vi "sushu-the first greater than 0 after less than 0.vi"(6 "Choose":string(combo)="Less", 7 "Direction":string(combo)="Forward", 8 "error out":errorcluster, 11 "Array In":dbl[](array[numeric])) -> (0 "error out 2":errorcluster)   [LabVIEW 2021]
panel:
  in  "OK":bool
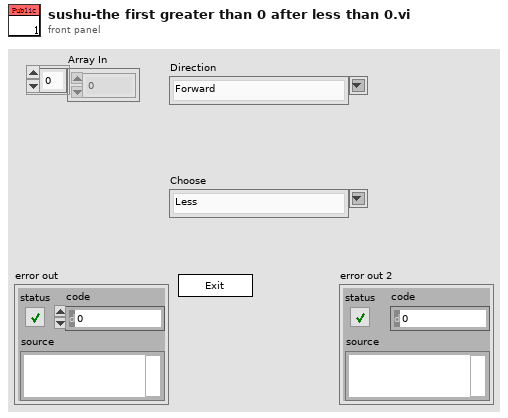
[diagram p1: front panel]
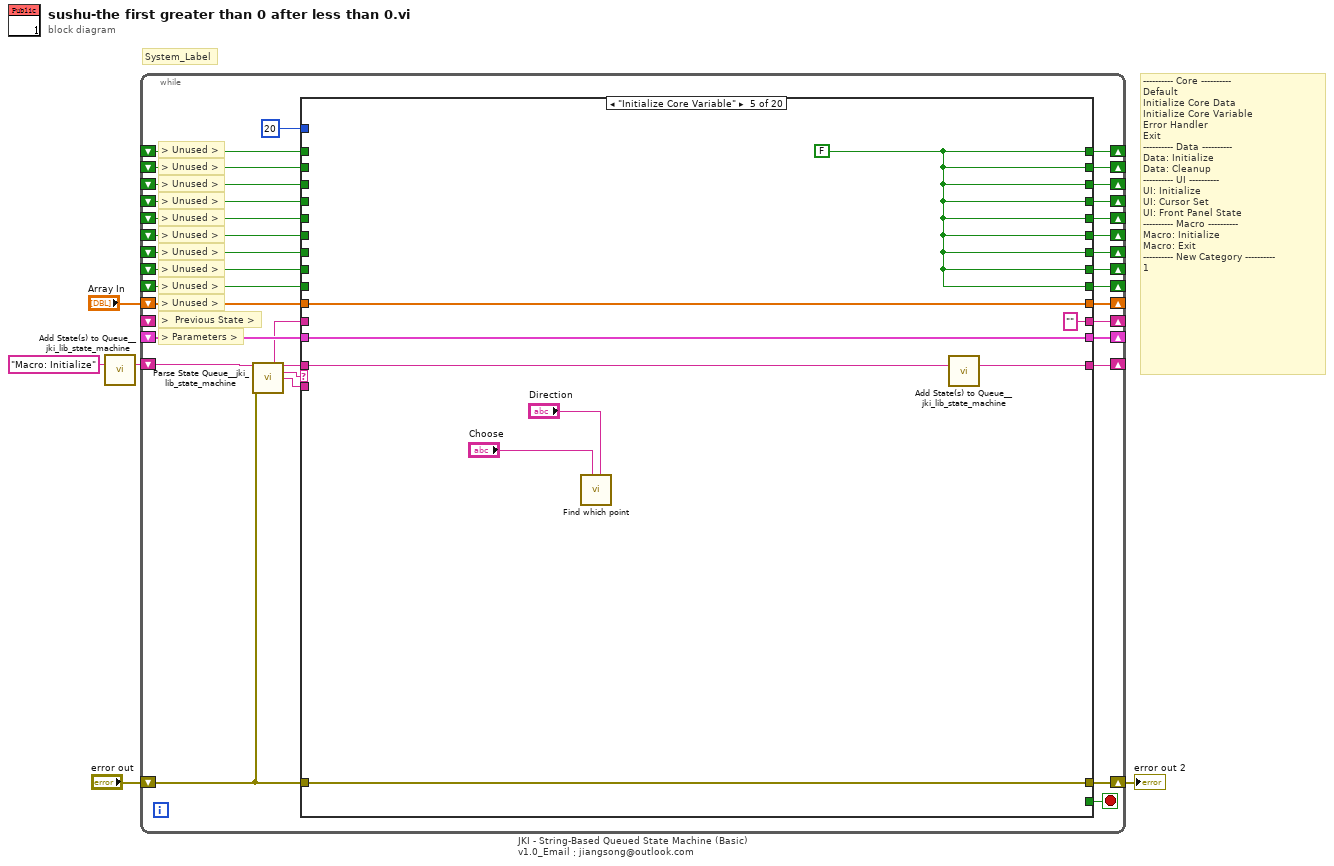
[diagram p0: block diagram]
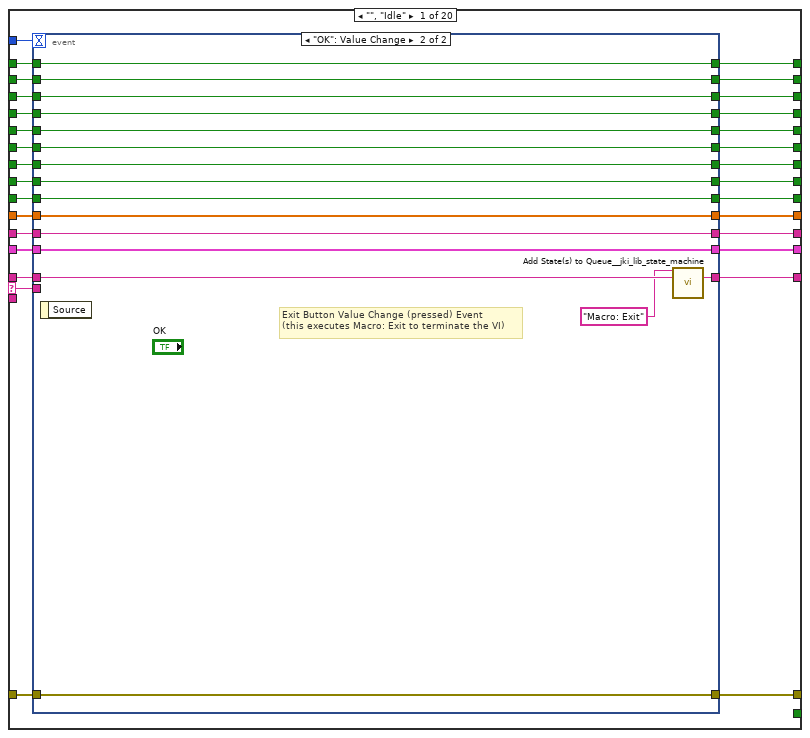
[diagram p2: hidden frame]
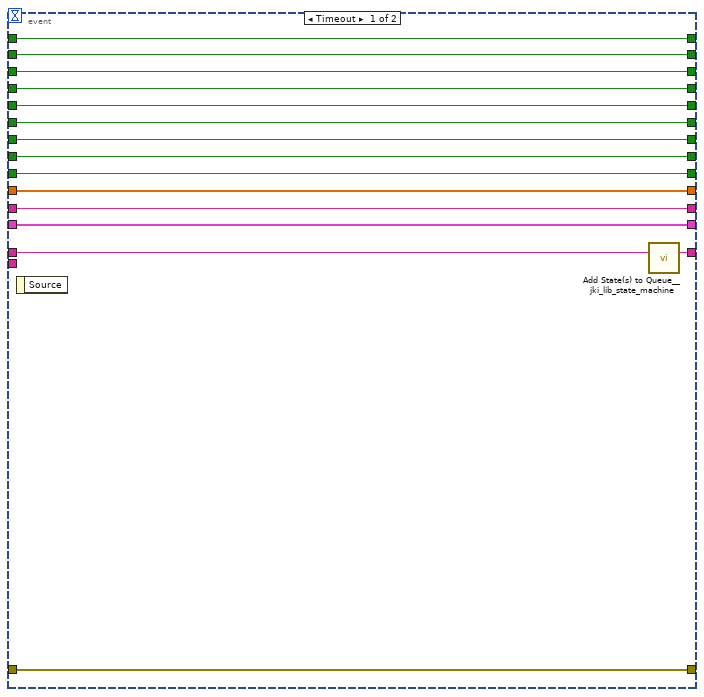
[diagram p3: hidden frame]
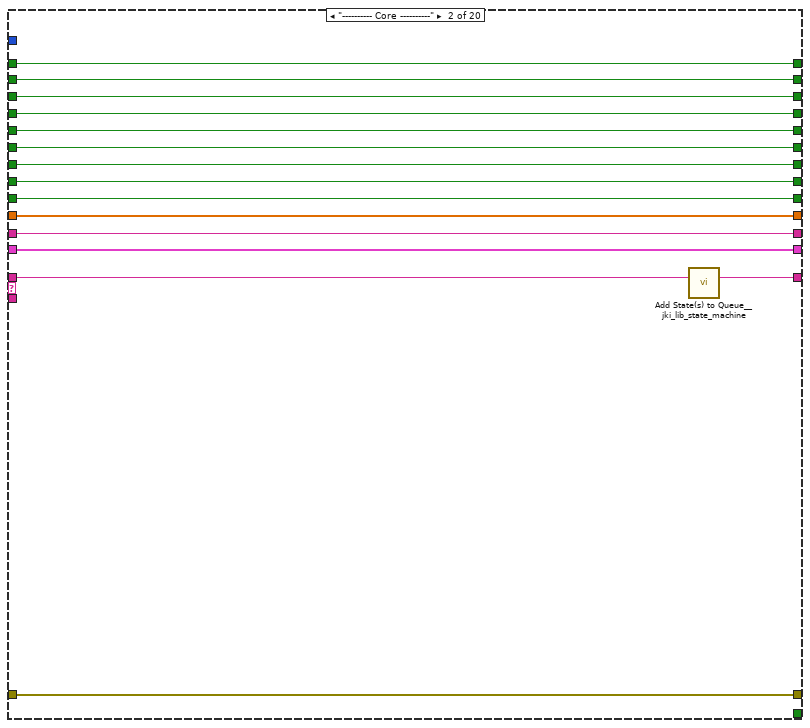
[diagram p4: hidden frame]
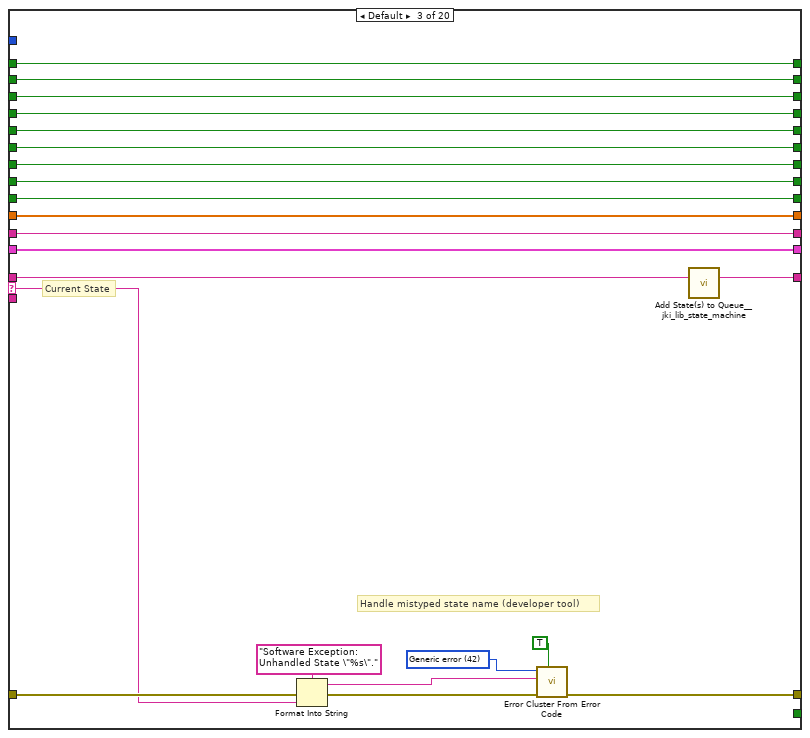
[diagram p5: hidden frame]
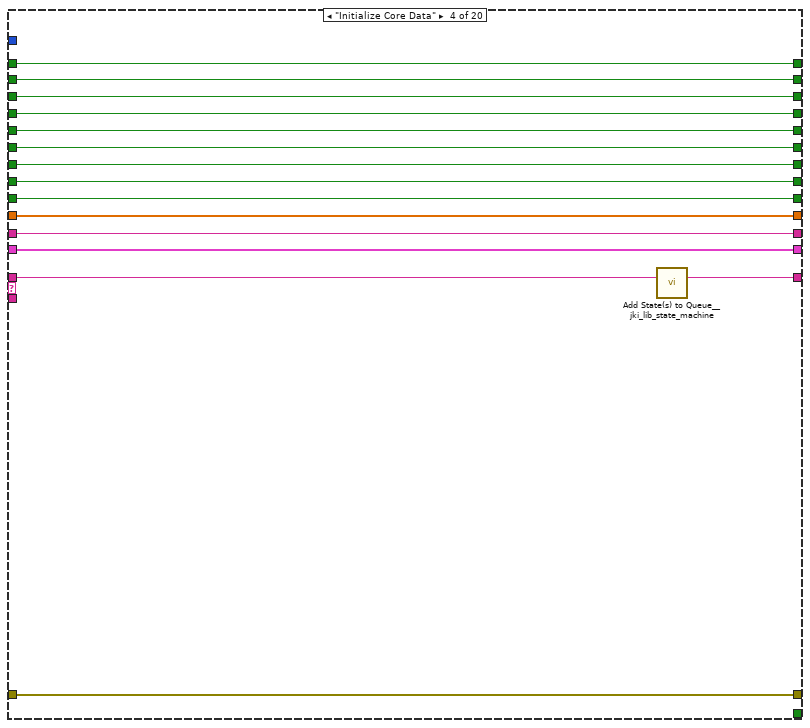
[diagram p6: hidden frame]
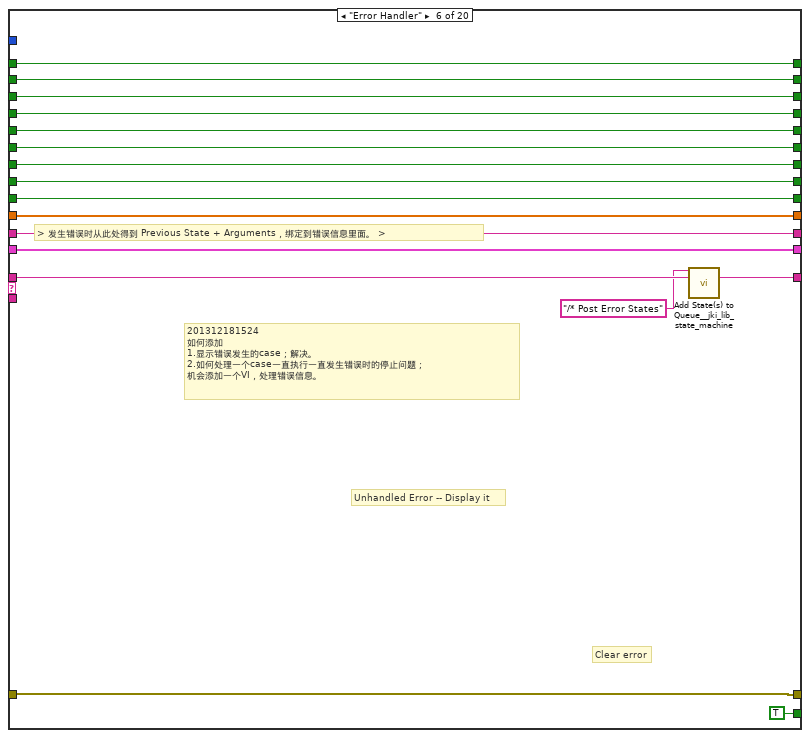
[diagram p7: hidden frame]
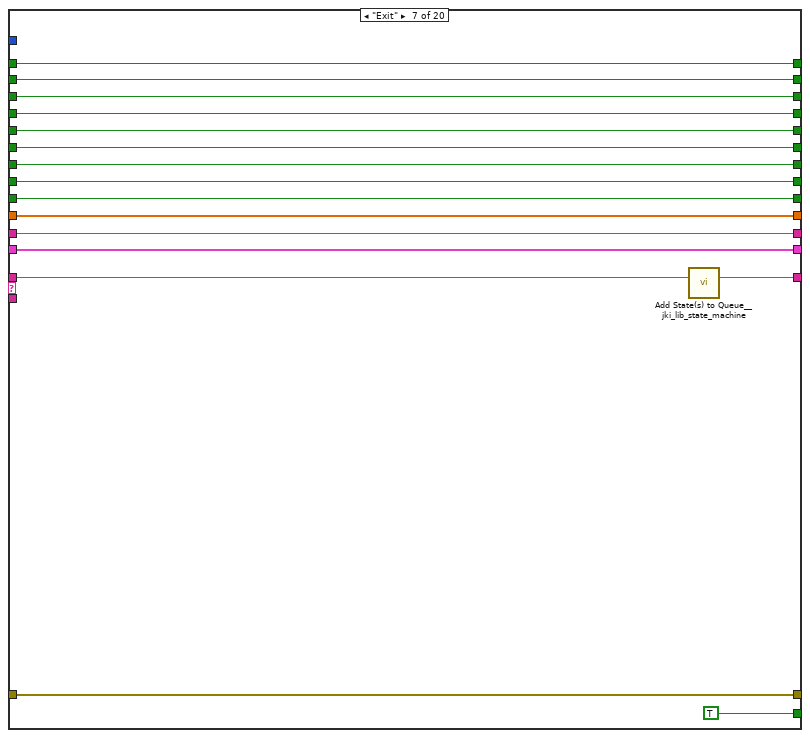
[diagram p8: hidden frame]
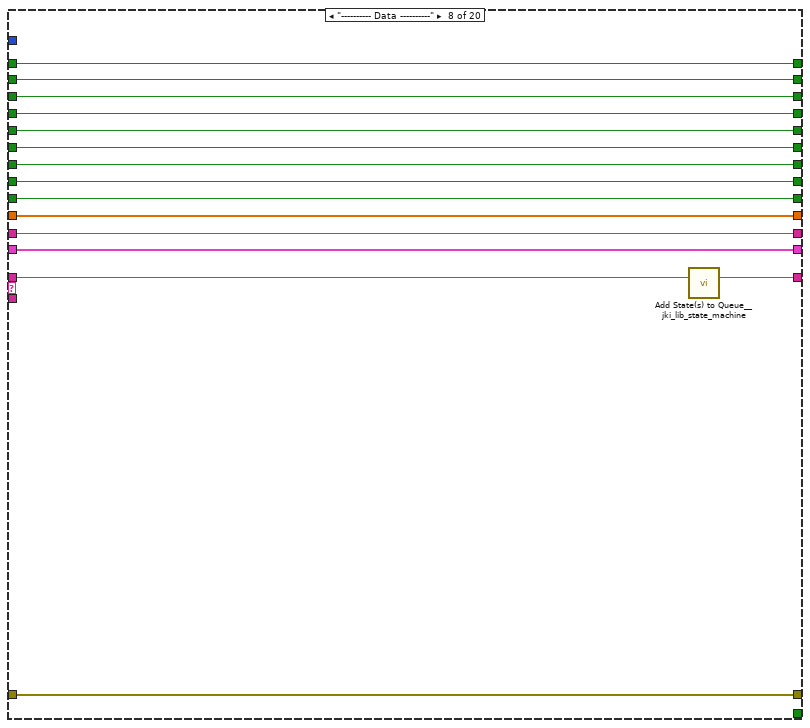
[diagram p9: hidden frame]
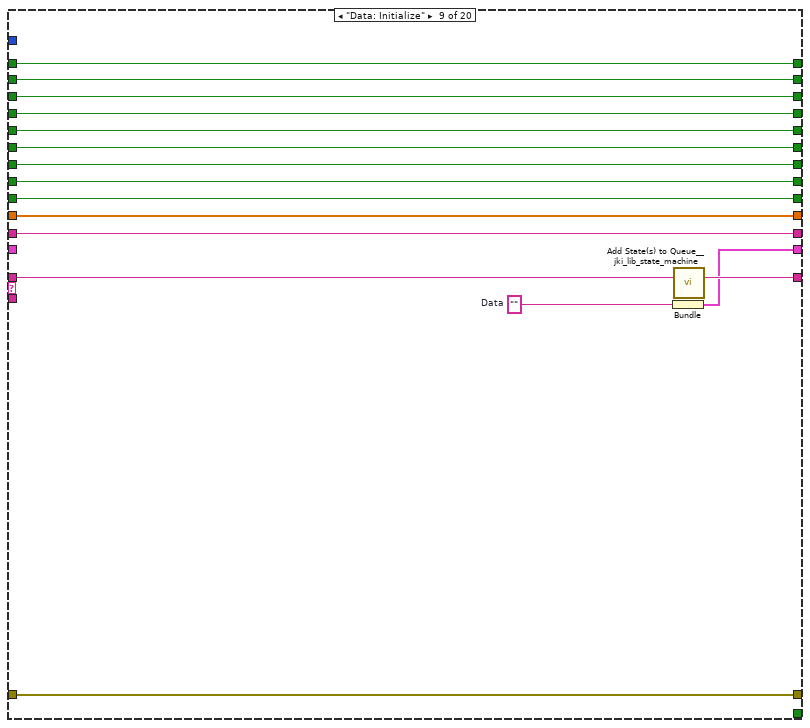
[diagram p10: hidden frame]
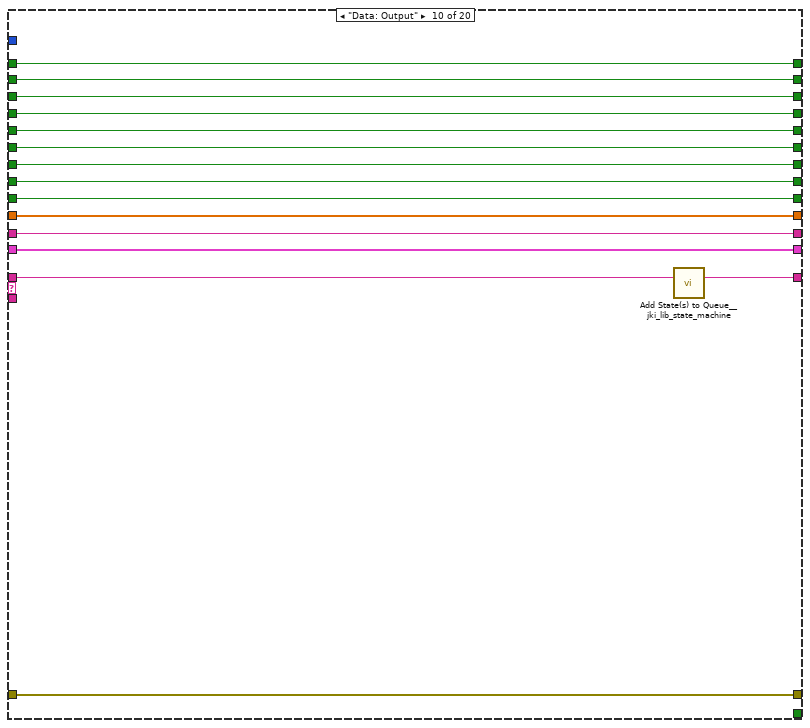
[diagram p11: hidden frame]
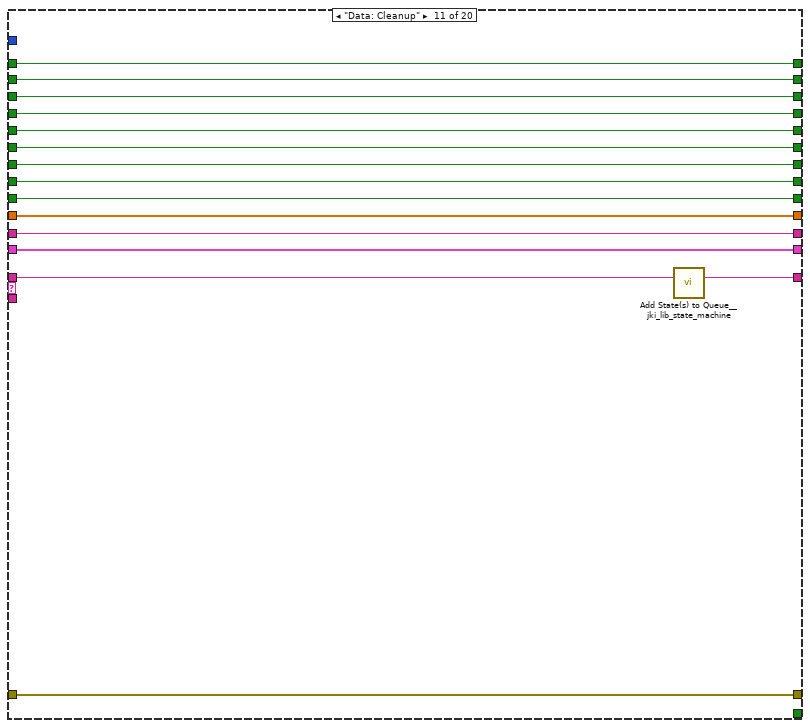
[diagram p12: hidden frame]
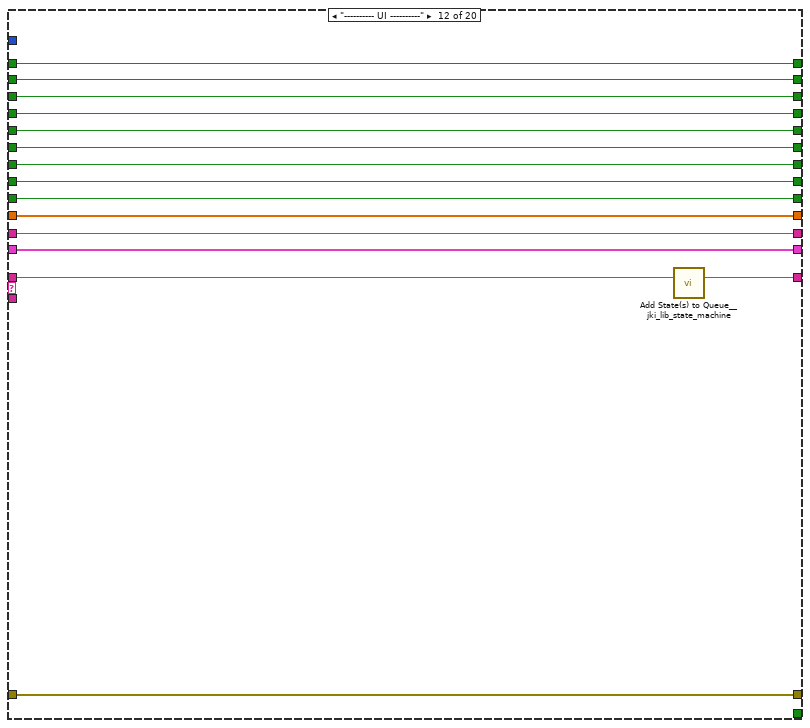
[diagram p13: hidden frame]
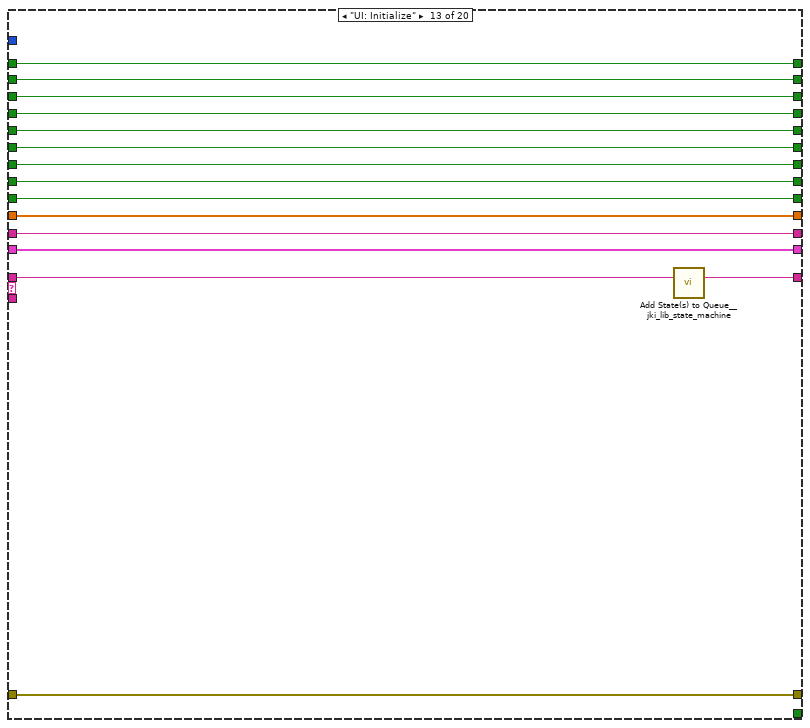
[diagram p14: hidden frame]
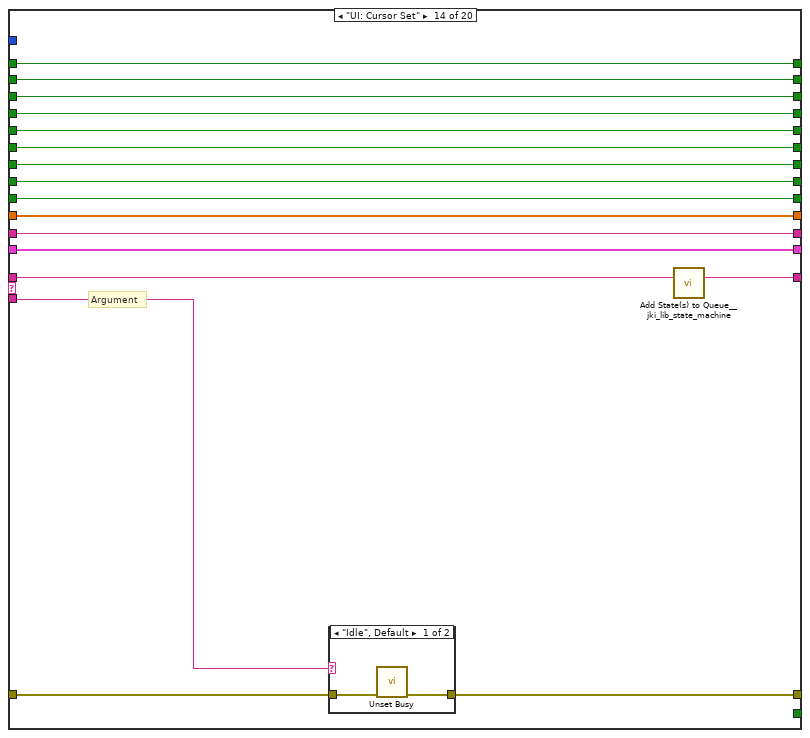
[diagram p15: hidden frame]
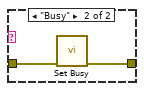
[diagram p16: hidden frame]
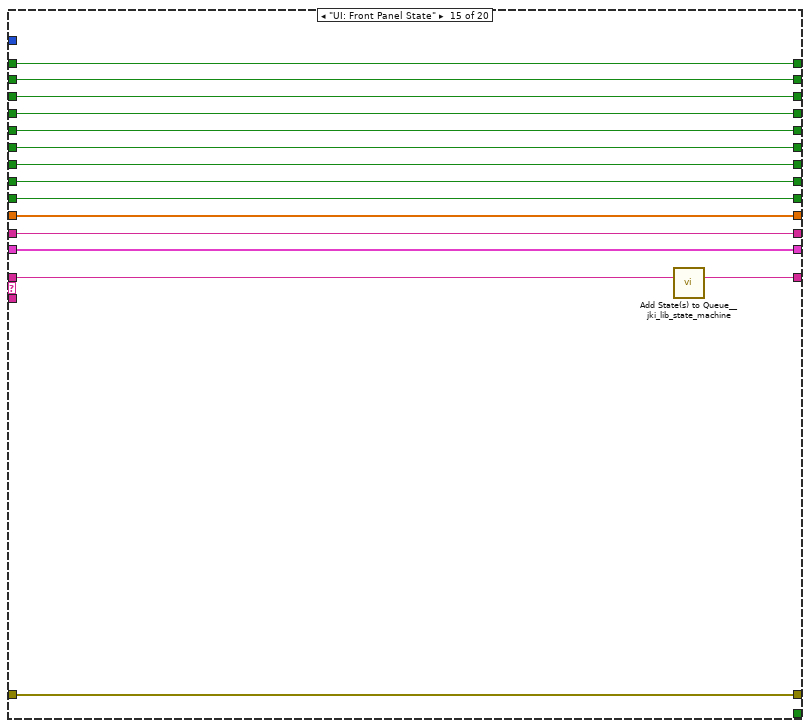
[diagram p17: hidden frame]
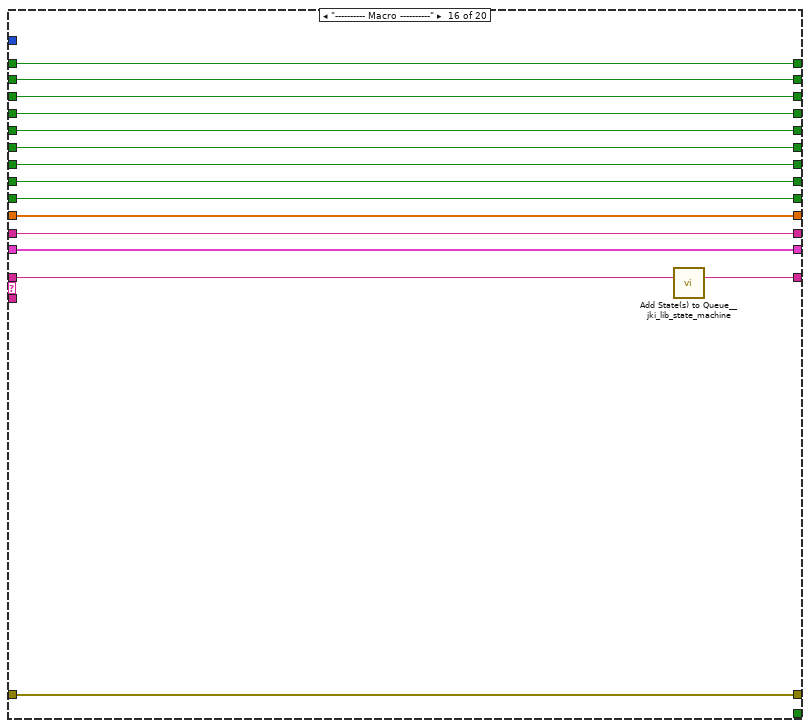
[diagram p18: hidden frame]
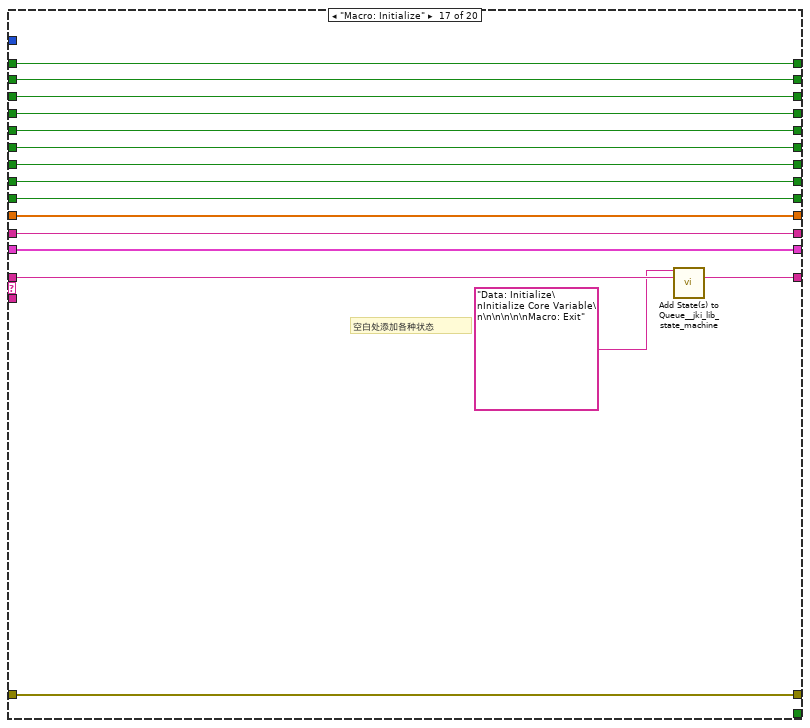
[diagram p19: hidden frame]
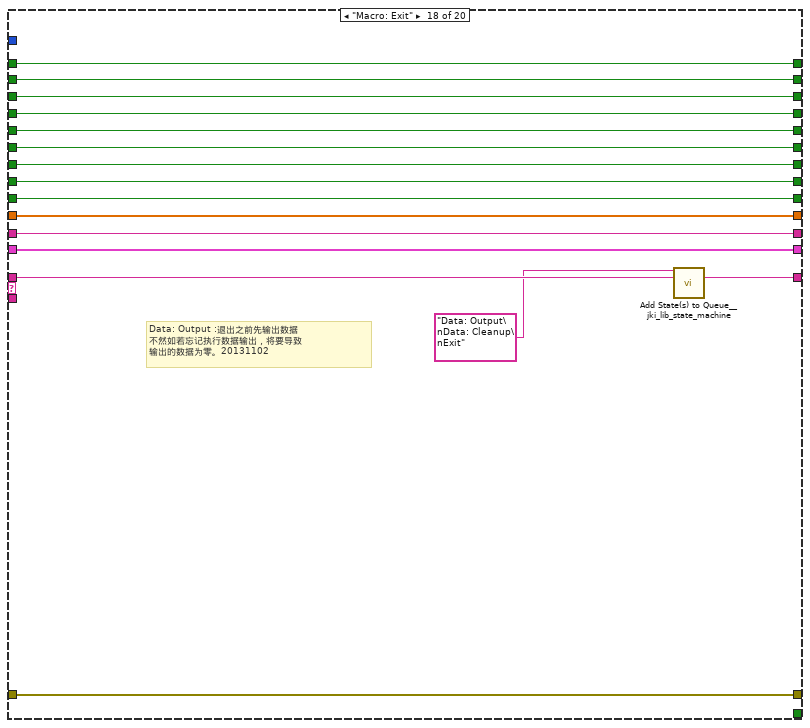
[diagram p20: hidden frame]
diagram:
  # "---------- Core ----------\nDefault\nInitialize Core Data\nInitialize Core Variable\nError Handler\nExit\n---------- Data ----------\nData: Initialize\nData: Cleanup\n---------- UI ----------\nUI: Initialize\nUI: Cursor Set\nUI: Front Panel State\n---------- Macro ----------\nMacro: Initialize\nMacro: Exit\n---------- New Category ----------\n1"
  # "System_Label"
  n1 = call <vilib>:"Add State(s) to Queue__jki_lib_state_machine.vi"("State(s) in (\"\")"="Macro: Initialize") -> ("States Out"=w3:string)  [unwired: 14 in]
  n2 = while "JKI - String-Based Queued State Machine (Basic) v1.0_Email：jiangsong@outlook.com" {
    shift-right: [w34] -> w5
    shift-left: "error out" -> [w30]
    shift-right: [w33] -> _
    shift-left: w3 -> [w35]
    shift-right: [w29] -> _
    shift-left: _ -> [w28]
    shift-right: [w16] -> _
    shift-left: _ -> [w24]
    shift-right: [w17] -> _
    shift-left: _ -> [w25]
    shift-right: [w18] -> _
    shift-left: _ -> [w26]
    shift-right: [w19] -> _
    shift-left: _ -> [w27]
    shift-right: [w12] -> _
    shift-left: _ -> [w20]
    shift-right: [w13] -> _
    shift-left: _ -> [w21]
    shift-right: [w14] -> _
    shift-left: _ -> [w22]
    shift-right: [w15] -> _
    shift-left: _ -> [w23]
    shift-right: [w7] -> _
    shift-left: _ -> [w10]
    shift-right: [w8] -> _
    shift-left: _ -> [_]
    shift-right: [w9] -> _
    shift-left: "Array In" -> [w11]
    stop <- w32 stop-if-true
    # "> Parameters >"
    # ">  Previous State >"
    # "> Unused >"
    # "> Unused >"
    # "> Unused >"
    # "> Unused >"
    # "> Unused >"
    # "> Unused >"
    # "> Unused >"
    # "> Unused >"
    # "> Unused >"
    # "> Unused >"
    n3 = call <vilib>:"Parse State Queue__jki_lib_state_machine.vi"("State Queue"=w35, "Error In (no error)"=w30) -> ("Previous State"=w6:string, "Remaining States"=w37:string, "Current State"=w38:string, "Arguments"=w36:string)  [unwired: 10 in]
    n4 = case shown="\"Initialize Core Variable\"" w38 {
      selector: w38 -> [w39 _ w115 _ _ _ _ _ _ _ _ _ _ _ _ _ _ _ _ _]
      tunnel: w37 -> [w68 w114 w136 w151 w160 w177 w193 w208 w224 w239 w254 w269 w284 w301 w320 w335 w351 w367 w382 w397]
      tunnel: w36 -> [_ _ _ _ _ _ _ _ _ _ _ _ _ w288 _ _ _ _ _ _]
      tunnel: [w66 w112 w116 w139 w158 w161 w179 w195 w212 w227 w241 w256 w271 w286 w307 w322 w338 w355 w370 w385] -> w34
      tunnel: w30 -> [w65 w112 w117 w139 w158 w161 w179 w195 w212 w227 w241 w256 w271 w287 w307 w322 w338 w355 w370 w385]
      tunnel: [w67 w113 w135 w150 w159 w176 w192 w207 w223 w238 w253 w268 w283 w300 w319 w334 w350 w366 w381 w396] -> w33
      tunnel: [_ _ _ _ _ TRUE TRUE _ _ _ _ _ _ _ _ _ _ _ _ _] -> w32
      tunnel: 20 ("Timeout") -> [w64 _ _ _ _ _ _ _ _ _ _ _ _ _ _ _ _ _ _ _]
      tunnel: [w63 w111 w134 w149 w154 w175 w191 w206 w222 w237 w252 w267 w282 w299 w318 w333 w349 w365 w380 w395] -> w29
      tunnel: w28 -> [w62 w111 w134 w149 _ w175 w191 w206 w222 w237 w252 w267 w282 w299 w318 w333 w349 w365 w380 w395]
      tunnel: w27 -> [w61 w110 w133 w148 _ w174 w190 w205 w221 w236 w251 w266 w281 w298 w317 w332 w348 w364 w379 w394]
      tunnel: w26 -> [w60 w109 w132 w147 _ w173 w189 w204 w220 w235 w250 w265 w280 w297 w316 w331 w347 w363 w378 w393]
      tunnel: w25 -> [w59 w108 w131 w146 _ w172 w188 w203 w219 w234 w249 w264 w279 w296 w315 w330 w346 w362 w377 w392]
      tunnel: w24 -> [w58 w107 w130 w145 _ w171 w187 w202 w218 w233 w248 w263 w278 w295 w314 w329 w345 w361 w376 w391]
      tunnel: w23 -> [w57 w106 w129 w144 _ w170 w186 w201 w217 w232 w247 w262 w277 w294 w313 w328 w344 w360 w375 w390]
      tunnel: w22 -> [w56 w105 w128 w143 _ w169 w185 w200 w216 w231 w246 w261 w276 w293 w312 w327 w343 w359 w374 w389]
      tunnel: w21 -> [w55 w104 w127 w142 _ w168 w184 w199 w215 w230 w245 w260 w275 w292 w311 w326 w342 w358 w373 w388]
      tunnel: w20 -> [w54 w103 w126 w141 _ w167 w183 w198 w214 w229 w244 w259 w274 w291 w310 w325 w341 w357 w372 w387]
      tunnel: [w53 w110 w133 w148 w154 w174 w190 w205 w221 w236 w251 w266 w281 w298 w317 w332 w348 w364 w379 w394] -> w19
      tunnel: [w52 w109 w132 w147 w154 w173 w189 w204 w220 w235 w250 w265 w280 w297 w316 w331 w347 w363 w378 w393] -> w18
      tunnel: [w51 w108 w131 w146 w154 w172 w188 w203 w219 w234 w249 w264 w279 w296 w315 w330 w346 w362 w377 w392] -> w17
      tunnel: [w50 w107 w130 w145 w154 w171 w187 w202 w218 w233 w248 w263 w278 w295 w314 w329 w345 w361 w376 w391] -> w16
      tunnel: [w49 w106 w129 w144 w154 w170 w186 w201 w217 w232 w247 w262 w277 w294 w313 w328 w344 w360 w375 w390] -> w15
      tunnel: [w48 w105 w128 w143 w154 w169 w185 w200 w216 w231 w246 w261 w276 w293 w312 w327 w343 w359 w374 w389] -> w14
      tunnel: [w47 w104 w127 w142 w154 w168 w184 w199 w215 w230 w245 w260 w275 w292 w311 w326 w342 w358 w373 w388] -> w13
      tunnel: [w46 w103 w126 w141 w154 w167 w183 w198 w214 w229 w244 w259 w274 w291 w310 w325 w341 w357 w372 w387] -> w12
      tunnel: w11 -> [w44 w102 w125 w140 w155 w166 w182 w197 w213 w228 w243 w258 w273 w290 w309 w324 w340 w356 w371 w386]
      tunnel: w6 -> [w42 w100 w124 w137 _ w163 w178 w194 w209 w225 w240 w255 w270 w285 w306 w321 w336 w352 w368 w383]
      tunnel: w10 -> [w40 w101 w123 w138 w157 w165 w181 w196 _ w226 w242 w257 w272 w289 w308 w323 w339 w354 w369 w384]
      tunnel: [w45 w102 w125 w140 w155 w166 w182 w197 w213 w228 w243 w258 w273 w290 w309 w324 w340 w356 w371 w386] -> w9
      tunnel: [w43 w100 w124 w137 "" ("Previous State + Arguments") w163 w178 w194 w209 w225 w240 w255 w270 w285 w306 w321 w336 w352 w368 w383] -> w8
      tunnel: [w41 w101 w123 w138 w157 w165 w181 w196 w211 w226 w242 w257 w272 w289 w308 w323 w339 w354 w369 w384] -> w7
      frame "", "Idle" {
        n5 = event shown="[1] \"OK\": Value Change" {
          selector: _ -> [_ _]
          dyn-events: _ -> [_ _]
          timeout: w64 -> [_ _]
          tunnel: w68 -> [w83 w99]
          tunnel: [w82 w98] -> w67
          tunnel: [w81 w97] -> w66
          tunnel: w65 -> [w81 w97]
          tunnel: [w80 w96] -> w63
          tunnel: w62 -> [w80 w96]
          tunnel: w61 -> [w79 w95]
          tunnel: w60 -> [w78 w94]
          tunnel: w59 -> [w77 w93]
          tunnel: w58 -> [w76 w92]
          tunnel: w57 -> [w75 w91]
          tunnel: w56 -> [w74 w90]
          tunnel: w55 -> [w73 w89]
          tunnel: w54 -> [w72 w88]
          tunnel: [w79 w95] -> w53
          tunnel: [w78 w94] -> w52
          tunnel: [w77 w93] -> w51
          tunnel: [w76 w92] -> w50
          tunnel: [w75 w91] -> w49
          tunnel: [w74 w90] -> w48
          tunnel: [w73 w89] -> w47
          tunnel: [w72 w88] -> w46
          tunnel: [w71 w87] -> w45
          tunnel: w44 -> [w71 w87]
          tunnel: [w69 w84] -> w43
          tunnel: w42 -> [w69 w84]
          tunnel: [w70 w86] -> w41
          tunnel: w40 -> [w70 w86]
          tunnel: w39 -> [_ _]
          event Timeout {
            n6 = event-data() -> ()  [unwired: 1 in, 1 out]
            n7 = call <vilib>:"Add State(s) to Queue__jki_lib_state_machine.vi"("State(s) in (\"\")"=w83) -> ("States Out"=w82:string)  [unwired: 14 in]
          }
          event "OK": Value Change {
            # "Exit Button Value Change (pressed) Event\n(this executes Macro: Exit to terminate the VI)"
            n8 = event-data() -> ()  [unwired: 1 in, 1 out]
            n9 = call <vilib>:"Add State(s) to Queue__jki_lib_state_machine.vi"("State(s) in Front (\"\")"="Macro: Exit", "State(s) in (\"\")"=w99) -> ("States Out"=w98:string)  [unwired: 13 in]
          }
        }
      }
      frame "---------- Core ----------" {
        # "Do not put any code in this frame.\n(it is a separator no-op)"
        n10 = call <vilib>:"Add State(s) to Queue__jki_lib_state_machine.vi"("State(s) in (\"\")"=w114) -> ("States Out"=w113:string)  [unwired: 14 in]
      }
      frame Default {
        w119 = 42 items=["No error", "Argument error", "Memory is full", "Out of zone", "End of file", "File already open", "Generic file I/O error", "File not found", "File permission error", "Disk is full", "Duplicate path", "Too many files open", "System feature not enabled", "Resource file not found", "Cannot add resource", "Resource not found", "Image not found", "Image memory error", "Pen does not exist", "Config type invalid", "Config token not found", "Config parse error", "Config memory error", "Bad external code format", "Bad external code offset", "External code not present", "Null window", "Destroy window error", "Null menu", "Print aborted", "Bad print record", "Print driver error", "Windows error during printing", "Memory error during printing", "Print dialog error", "Generic print error", "Invalid device refnum", "Device not found", "Device parameter error", "Device unit error", "Cannot open device", "Device call aborted", "Generic error", "Cancelled by user", "Object ID too low", "Object ID too high", "Object not in heap", "Unknown heap", "Unknown object (invalid DefProc)", "Unknown object (DefProc not in table)", "Message out of range", "Invalid (null) method", "Unknown message", "Manager call not supported", "Bad address", "Network operation in progress", "Network operation timed out", "Connection is busy", "Network attribute not supported", "Network error", "Address in use", "System out of memory", "Connection aborted", "Connection refused", "Not connected", "Already connected", "Connection closed", "Initialization error (interapplication manager)", "Bad occurrence", "Wait on unbound occurrence handler", "Occurrence queue overflow", "Datalog type conflict", "Unused", "Unrecognized type (interapplication manager)", "Memory corrupt", "Failed to make temporary DLL", "Old CIN version", "Drag socket not found", "Failed to load drop-object", "Failed to register OLE object", "Failed to release OLE object", "Format specifier type mismatch", "Unknown format specifier", "Too few format specifiers", "Too many format specifiers", "Scan failed", "Newer CIN version", "Error converting to variant", "Runtime menu error", "Password tampered", "Variant attribute not found", "Incompatible variant data type", "Event data is not available", "Event Store is not present", "Occurrence is not found", "Event Queue is not created", "Event info is not available", "Refnum passed is NULL", "Error retrieving Class GUID", "Error retrieving CoClass GUID", "Error retrieving TypeLib GUID.", "Bad built application magic bytes.", "Specific driver is different from the specific driver associated with the Logical Name.", "There is no session opened to the class driver.", "Max Error", "MAX - Error with config objects", "MAX - Error loading configuration", "MAX - Group not supported"]
        # "Current State"
        # "Handle mistyped state name (developer tool)"
        # "Do not delete, rename, or modify this frame.\n(this is used to capture unhandled states and typos)"
        n11 = Format Into String(format string="Software Exception: Unhandled State \"%s\"." ("message"), error in=w117, w115) -> (resulting string=w120:string, error out=w121:errorcluster)  [unwired: 1 in]
        n12 = call <vilib>:"Error Cluster From Error Code.vi"("show call chain? (False)"=TRUE, "error in (no error)"=w121, "error message (\"\")"=w120, "error code (0)"=w119) -> ("error out"=w116:errorcluster)  [unwired: 5 in]
        n13 = call <vilib>:"Add State(s) to Queue__jki_lib_state_machine.vi"("State(s) in (\"\")"=w136) -> ("States Out"=w135:string)  [unwired: 14 in]
      }
      frame "Initialize Core Data" {
        # "Do not delete, rename, or modify this frame.\n(this is used to determine panel behavior on exit)"
        n14 = call <vilib>:"Add State(s) to Queue__jki_lib_state_machine.vi"("State(s) in (\"\")"=w151) -> ("States Out"=w150:string)  [unwired: 14 in]
      }
      frame "Initialize Core Variable" {
        w154 = FALSE
        n15 = call <userlib>:"Find which point.vi"("Direction"="Direction", "Choose"="Choose") -> ()  [unwired: 9 in, 1 out]
        n16 = call <vilib>:"Add State(s) to Queue__jki_lib_state_machine.vi"("State(s) in (\"\")"=w160) -> ("States Out"=w159:string)  [unwired: 14 in]
      }
      frame "Error Handler" {
        # "> 发生错误时从此处得到 Previous State + Arguments，绑定到错误信息里面。 >"
        # "201312181524\n如何添加\n1.显示错误发生的case；解决。\n2.如何处理一个case一直执行一直发生错误时的停止问题；\n机会添加一个VI，处理错误信息。"
        # "Clear error"
        # "Unhandled Error -- Display it"
        # "Handle any errors here.\nYou can also output any states to clean-up after errors occur"
        n17 = call <vilib>:"Add State(s) to Queue__jki_lib_state_machine.vi"("State(s) in Front (\"\")"="/* Post Error States", "State(s) in (\"\")"=w177) -> ("States Out"=w176:string)  [unwired: 13 in]
      }
      frame "Exit" {
        # "Do not put any code in this frame.\n(No errors that occur here will be handled.)"
        n18 = call <vilib>:"Add State(s) to Queue__jki_lib_state_machine.vi"("State(s) in (\"\")"=w193) -> ("States Out"=w192:string)  [unwired: 14 in]
      }
      frame "---------- Data ----------" {
        # "Do not put any code in this frame.\n(It is a separator no-op. You can make a copy of this frame to create a new Data frame)"
        n19 = call <vilib>:"Add State(s) to Queue__jki_lib_state_machine.vi"("State(s) in (\"\")"=w208) -> ("States Out"=w207:string)  [unwired: 14 in]
      }
      frame "Data: Initialize" {
        w210 = ""  # Data
        # "Initialize the shift-register data, here.\n(data names are defined by what you wire into the bundle function)"
        n20 = Bundle("Data"=w210) -> (w211:cluster{"Data":string})  [unwired: 1 in]
        n21 = call <vilib>:"Add State(s) to Queue__jki_lib_state_machine.vi"("State(s) in (\"\")"=w224) -> ("States Out"=w223:string)  [unwired: 14 in]
      }
      frame "Data: Output" {
        # "(退出此VI之前，输出程序中的变量的最终结果，必须在这里输出最终数据)"
        n22 = call <vilib>:"Add State(s) to Queue__jki_lib_state_machine.vi"("State(s) in (\"\")"=w239) -> ("States Out"=w238:string)  [unwired: 14 in]
      }
      frame "Data: Cleanup" {
        # "Cleanup any data and references, here.\n(this is called automatically, by the Macro: Exit)"
        n23 = call <vilib>:"Add State(s) to Queue__jki_lib_state_machine.vi"("State(s) in (\"\")"=w254) -> ("States Out"=w253:string)  [unwired: 14 in]
      }
      frame "---------- UI ----------" {
        # "Do not put any code in this frame.\n(It is a separator no-op. You can make a copy of this frame to create a new UI frame)"
        n24 = call <vilib>:"Add State(s) to Queue__jki_lib_state_machine.vi"("State(s) in (\"\")"=w269) -> ("States Out"=w268:string)  [unwired: 14 in]
      }
      frame "UI: Initialize" {
        # "Initialize the User Interface, here.\n(this is called automatically, by the Macro: Init)"
        n25 = call <vilib>:"Add State(s) to Queue__jki_lib_state_machine.vi"("State(s) in (\"\")"=w284) -> ("States Out"=w283:string)  [unwired: 14 in]
      }
      frame "UI: Cursor Set" {
        # "Argument"
        # "Set and Unset Cursor Busy.\n(Usage: \"UI: Cursor Set >> Busy|Idle\")"
        n26 = case shown="\"Idle\", Default" w288 {
          tunnel: w287 -> [w303 w305]
          tunnel: [w302 w304] -> w286
          frame "Idle", Default {
            n27 = call <vilib>:"Unset Busy.vi"("error in (no error)"=w303) -> ("error out"=w302:errorcluster)  [unwired: 10 in]
          }
          frame "Busy" {
            n28 = call <vilib>:"Set Busy.vi"("error in (no error)"=w305) -> ("error out"=w304:errorcluster)  [unwired: 9 in, 1 out]
          }
        }
        n29 = call <vilib>:"Add State(s) to Queue__jki_lib_state_machine.vi"("State(s) in (\"\")"=w301) -> ("States Out"=w300:string)  [unwired: 14 in]
      }
      frame "UI: Front Panel State" {
        # "Set Front Panel Open or Closed\n(Usage: \"UI: Front Panel State >> Open|Close\")"
        n30 = call <vilib>:"Add State(s) to Queue__jki_lib_state_machine.vi"("State(s) in (\"\")"=w320) -> ("States Out"=w319:string)  [unwired: 14 in]
      }
      frame "---------- Macro ----------" {
        # "Do not put any code in this frame.\n(It is a separator no-op. You can make a copy of this frame to create a new Macro frame)"
        n31 = call <vilib>:"Add State(s) to Queue__jki_lib_state_machine.vi"("State(s) in (\"\")"=w335) -> ("States Out"=w334:string)  [unwired: 14 in]
      }
      frame "Macro: Initialize" {
        # "空白处添加各种状态"
        # "Initialization Macro\n(This is called once, when the VI starts)"
        n32 = call <vilib>:"Add State(s) to Queue__jki_lib_state_machine.vi"("State(s) in Front (\"\")"="Data: Initialize\nInitialize Core Variable\n\n\n\n\n\nMacro: Exit", "State(s) in (\"\")"=w351) -> ("States Out"=w350:string)  [unwired: 13 in]
      }
      frame "Macro: Exit" {
        # "Data: Output :退出之前先输出数据\n不然如若忘记执行数据输出，将要导致\n输出的数据为零。20131102"
        # "Exit Macro\n(This is called once, when the VI exits)"
        n33 = call <vilib>:"Add State(s) to Queue__jki_lib_state_machine.vi"("State(s) in Front (\"\")"="Data: Output\nData: Cleanup\nExit", "State(s) in (\"\")"=w367) -> ("States Out"=w366:string)  [unwired: 13 in]
      }
      frame "---------- New Category ----------" {
        # "Template Separator\n(You can make a copy of, or modify, this frame)"
        n34 = call <vilib>:"Add State(s) to Queue__jki_lib_state_machine.vi"("State(s) in (\"\")"=w382) -> ("States Out"=w381:string)  [unwired: 14 in]
      }
      frame "1" {
        # "Your code here.\n(You can make a copy of, or modify, this frame)"
        n35 = call <vilib>:"Add State(s) to Queue__jki_lib_state_machine.vi"("State(s) in (\"\")"=w397) -> ("States Out"=w396:string)  [unwired: 14 in]
      }
    }
  }
  "error out 2" <- w5
